vi "S_WriteClassAttribute.vi"(0 "reference in":refnum<class "SubTemplate.lvclass">, 5 "Error In":errorcluster) -> (14 "reference out":refnum<class "SubTemplate.lvclass">, 19 "Error Out":errorcluster)   [LabVIEW 2020]
uses:
  SubTemplate.lvclass
  BaseTemplate/protected/ClassAttributes.ctl
  BaseTemplate/BaseTemplate.lvclass
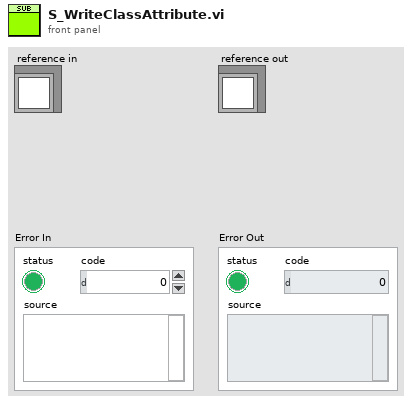
[diagram p1: front panel]
types:
  T1 = typedef "BaseTemplate.lvclass/ClassAttributes.ctl" = cluster{"classAttribute1":bool}
  T2 = typedef "SubTemplate.lvclass/ClassAttributes.ctl" = cluster{"Base class":T1}
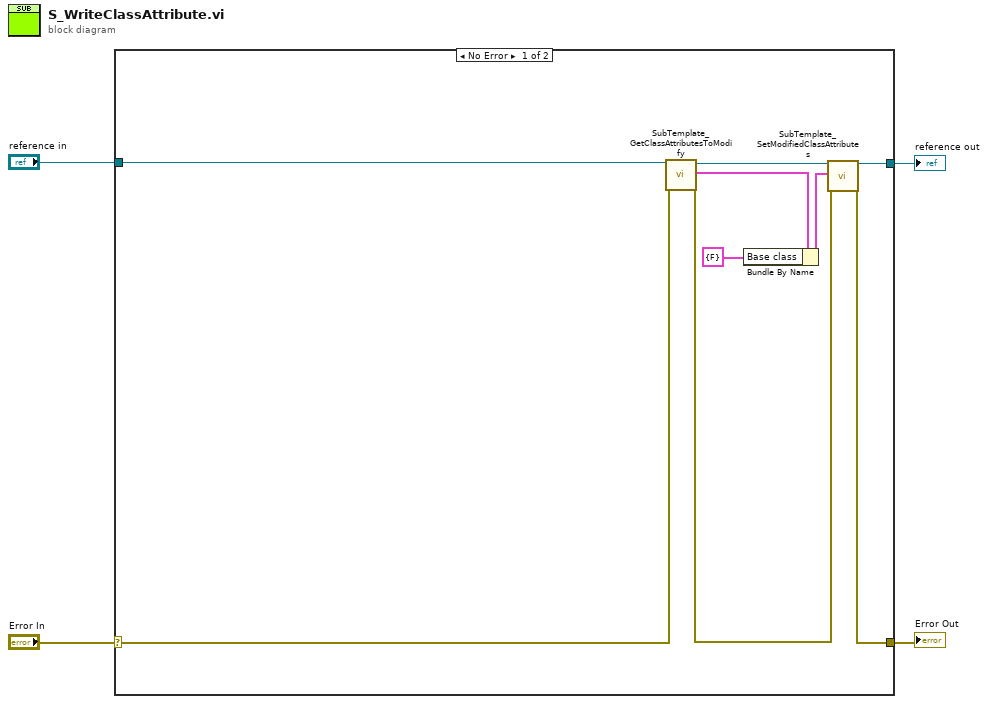
[diagram p0: block diagram]
diagram:
  n1 = case shown="No Error" "Error In" {
    selector: "Error In" -> [w7 w15]
    tunnel: [w10 w15] -> w3
    tunnel: [w9 w14] -> w1
    tunnel: "reference in" -> [w6 w14]
    frame No Error {
      n2 = call "SubTemplate_GetClassAttributesToModify.vi"("reference in"=w6, "error in (no error)"=w7) -> ("reference out"=w11:refnum<class "SubTemplate.lvclass">, "Class attributes"=w13:T2, "error out"=w8:errorcluster)  [unwired: 14 in, 1 out]
      n3 = Bundle By Name(cluster=w13, "Base class"=T1 {"classAttribute1"=FALSE}) -> (w12:T2)
      n4 = call "SubTemplate_SetModifiedClassAttributes.vi"("reference in"=w11, "Class attributes"=w12, "error in (no error)"=w8) -> ("reference out"=w9:refnum<class "SubTemplate.lvclass">, "error out"=w10:errorcluster)  [unwired: 15 in]
    }
    frame Error {
    }
  }
  "Error Out" <- w3
  "reference out" <- w1
